vi "Support instrTrayIcon_test.vi"() -> ()   [LabVIEW 2018]
panel:
  out "decimal integer string":string
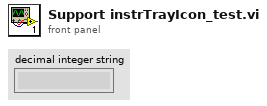
[diagram p1: front panel]
types:
  T1 = enum16{"open", "replace", "create", "open or create", "replace or create", "replace or create with confirmation"}
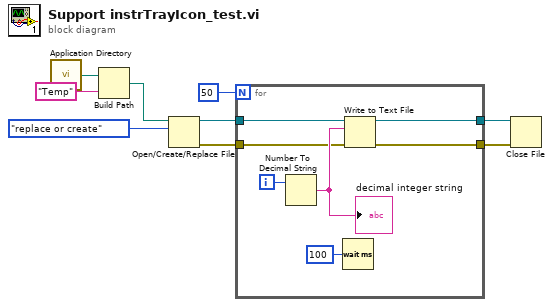
[diagram p0: block diagram]
diagram:
  n1 = call <vilib>:"Application Directory.vi"() -> ("Application Directory"=w9:path)
  n2 = Build Path(base path=w9, name or relative path="Temp") -> (appended path=w7:path)
  n3 = Open/Create/Replace File(file path (use dialog)=w7, operation (0:open)=T1."replace or create") -> (refnum out=w5:refnum<file>, error out=w3:errorcluster)  [unwired: 4 in, 1 out]
  n4 = for {
    N: 50 -> [_]
    tunnel: w5 -> [w16]
    tunnel: [w14] -> w2
    tunnel: w3 -> [w11]
    tunnel: [w10] -> w1
    i -> [w13]
    n5 = Number To Decimal String(number=w13) -> (decimal integer string=w12:string)  [unwired: 1 in]
    "decimal integer string" <- w12
    n6 = Wait (ms)(milliseconds to wait=u32 100) -> ()  [unwired: 1 out]
    n7 = Write to Text File(file (use dialog)=w16, text=w12, error in=w11) -> (refnum out=w14:refnum<file>, error out=w10:errorcluster)  [unwired: 1 in, 1 out]
  }
  n8 = Close File(refnum=w2, error in=w1) -> ()  [unwired: 2 out]
